vi "Generate Custom Error.vi"(8 "error in":errorcluster, 10 "PAR1":string, 11 "GOLPI error":T1) -> (0 "error out":errorcluster)   [LabVIEW 2020, in "GOLPI library.lvlib"]
doc: "Generate custom error of the GOLPI library. Some errors has input parameters (PAR1) to provide more detailed description."
uses:
  GOLPI library.lvlib
  Type Definitions/Custom Error Codes Enum Type Def.vi
  <vilib>/Utility/error.llb/Error Cluster From Error Code.vi
  <vilib>/ErrorRing/Error Ring.xnode
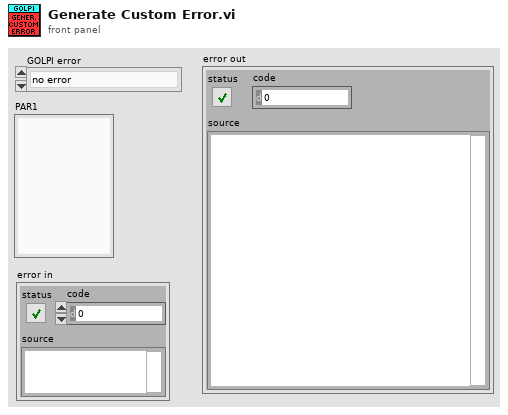
[diagram p1: front panel]
types:
  T1 = typedef "GOLPI library.lvlib/Custom Error Codes Enum Type Def.vi" = enum16{"no error", "00 working directory PAR1 missing", "01 octave binary PAR1 missing", "02 octave report error PAR1", "03 empty output last cmd PAR1", "04 missing temporary file PAR1", "05 pwd PAR 1 not exist", "06 oct package not installed", "07 octave default binary missing", "10 var PAR1 not string, vect", "11 var PAR1 not num, scal, ~compl", "12 var PAR1 not num, scal, compl", "13 var PAR1 not num, vect, ~compl", "14 var PAR1 not num, vect, compl", "15 var PAR1 not num, mat, ~compl", "16 var PAR1 not num, mat, ~compl", "30 read timeout", "60 bitstream transport failed", "61 bitstream decode error PAR1", "62 bitstream cannot be set", "70 struct transfer not possible", "80 struct: cluster elem. PAR1 not implem.", "81 struct: structure field PAR1 not implem.", "82 struct: size mismatch of PAR1", "83 struct: type mismatch of PAR1", "98 internal error", "99 not finished", "90 Not supported in Matlab mode", "91 Matlab variable transfer error", "92 Matlab Script Error", "100 Variable Pipe Mode cannot be set"}
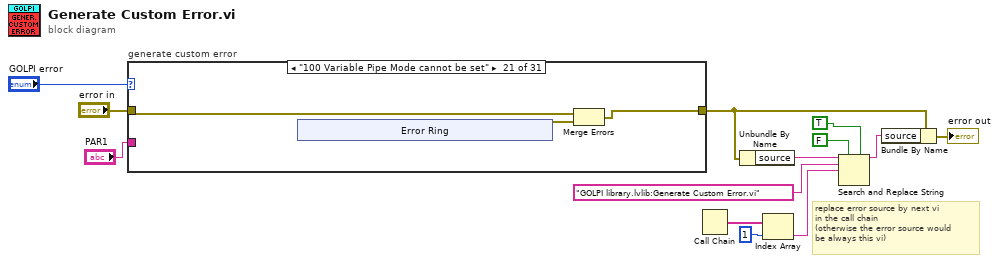
[diagram p0: block diagram]
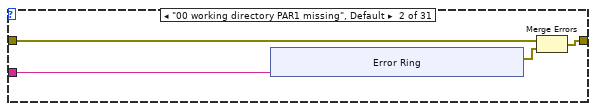
[diagram p3: hidden frame]
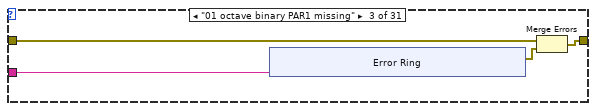
[diagram p4: hidden frame]
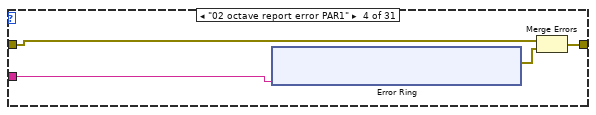
[diagram p5: hidden frame]
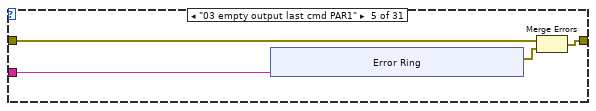
[diagram p6: hidden frame]
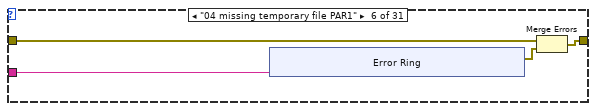
[diagram p7: hidden frame]
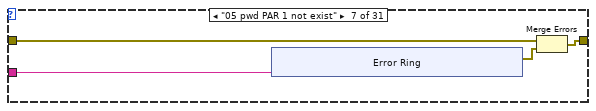
[diagram p8: hidden frame]
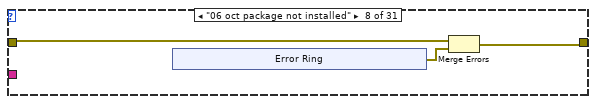
[diagram p9: hidden frame]
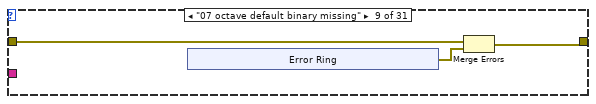
[diagram p10: hidden frame]
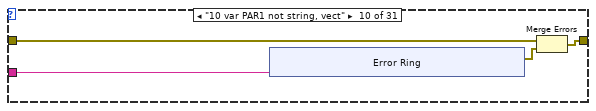
[diagram p11: hidden frame]
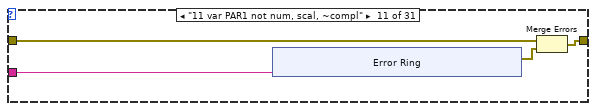
[diagram p12: hidden frame]
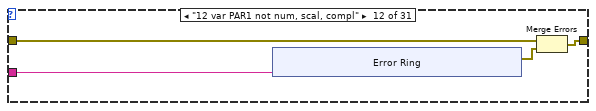
[diagram p13: hidden frame]
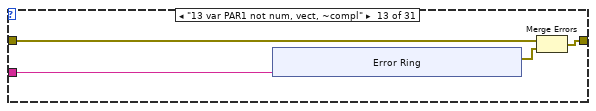
[diagram p14: hidden frame]
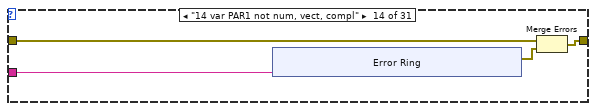
[diagram p15: hidden frame]
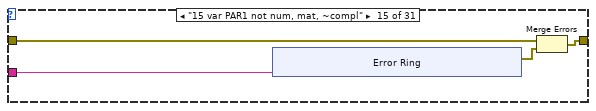
[diagram p16: hidden frame]
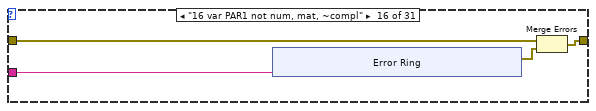
[diagram p17: hidden frame]
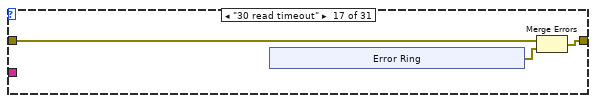
[diagram p18: hidden frame]
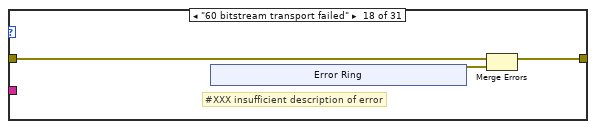
[diagram p19: hidden frame]
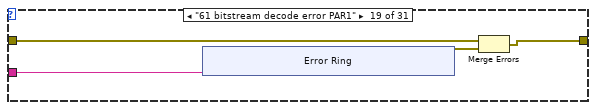
[diagram p20: hidden frame]
diagram:
  # "replace error source by next vi\nin the call chain\n(otherwise the error source would\nbe always this vi)"
  n1 = case "generate custom error" shown="\"100 Variable Pipe Mode cannot be set\"" "GOLPI error" {
    tunnel: "PAR1" -> [_ w18 w29 w38 w51 w59 w70 _ _ w97 w108 w120 w130 w142 w152 w163 _ _ w191 _ _ _ w225 w236 w247 w258 _ w277 w288 _ _]
    tunnel: [w14 w16 w27 w37 w48 w60 w71 w82 w89 w98 w109 w119 w132 w141 w153 w164 w174 w182 w192 w201 w209 w217 w226 w238 w249 w260 w270 w279 w290 w300 w307] -> w7
    tunnel: "error in" -> [w14 w15 w26 w39 w49 w61 w72 w81 w90 w99 w110 w122 w133 w143 w154 w165 w175 w183 w190 w202 w210 w218 w227 w237 w248 w259 w269 w278 w289 w299 w308]
    frame "no error" {
    }
    frame "00 working directory PAR1 missing", Default {
      n2 = xnode "Error Ring"("parameter 0"=w18) -> ("error out"=w17:errorcluster)
      n3 = Merge Errors(w15, w17) -> (w16:errorcluster)
    }
    frame "01 octave binary PAR1 missing" {
      n4 = xnode "Error Ring"("parameter 0"=w29) -> ("error out"=w28:errorcluster)
      n5 = Merge Errors(w26, w28) -> (w27:errorcluster)
    }
    frame "02 octave report error PAR1" {
      n6 = xnode "Error Ring"("parameter 0"=w38) -> ("error out"=w40:errorcluster)
      n7 = Merge Errors(w39, w40) -> (w37:errorcluster)
    }
    frame "03 empty output last cmd PAR1" {
      n8 = xnode "Error Ring"("parameter 0"=w51) -> ("error out"=w50:errorcluster)
      n9 = Merge Errors(w49, w50) -> (w48:errorcluster)
    }
    frame "04 missing temporary file PAR1" {
      n10 = xnode "Error Ring"("parameter 0"=w59) -> ("error out"=w62:errorcluster)
      n11 = Merge Errors(w61, w62) -> (w60:errorcluster)
    }
    frame "05 pwd PAR 1 not exist" {
      n12 = xnode "Error Ring"("parameter 0"=w70) -> ("error out"=w73:errorcluster)
      n13 = Merge Errors(w72, w73) -> (w71:errorcluster)
    }
    frame "06 oct package not installed" {
      n14 = xnode "Error Ring"() -> ("error out"=w83:errorcluster)
      n15 = Merge Errors(w81, w83) -> (w82:errorcluster)
    }
    frame "07 octave default binary missing" {
      n16 = xnode "Error Ring"() -> ("error out"=w91:errorcluster)
      n17 = Merge Errors(w90, w91) -> (w89:errorcluster)
    }
    frame "10 var PAR1 not string, vect" {
      n18 = xnode "Error Ring"("parameter 0"=w97) -> ("error out"=w100:errorcluster)
      n19 = Merge Errors(w99, w100) -> (w98:errorcluster)
    }
    frame "11 var PAR1 not num, scal, ~compl" {
      n20 = xnode "Error Ring"("parameter 0"=w108) -> ("error out"=w111:errorcluster)
      n21 = Merge Errors(w110, w111) -> (w109:errorcluster)
    }
    frame "12 var PAR1 not num, scal, compl" {
      n22 = xnode "Error Ring"("parameter 0"=w120) -> ("error out"=w121:errorcluster)
      n23 = Merge Errors(w122, w121) -> (w119:errorcluster)
    }
    frame "13 var PAR1 not num, vect, ~compl" {
      n24 = xnode "Error Ring"("parameter 0"=w130) -> ("error out"=w131:errorcluster)
      n25 = Merge Errors(w133, w131) -> (w132:errorcluster)
    }
    frame "14 var PAR1 not num, vect, compl" {
      n26 = xnode "Error Ring"("parameter 0"=w142) -> ("error out"=w144:errorcluster)
      n27 = Merge Errors(w143, w144) -> (w141:errorcluster)
    }
    frame "15 var PAR1 not num, mat, ~compl" {
      n28 = xnode "Error Ring"("parameter 0"=w152) -> ("error out"=w155:errorcluster)
      n29 = Merge Errors(w154, w155) -> (w153:errorcluster)
    }
    frame "16 var PAR1 not num, mat, ~compl" {
      n30 = xnode "Error Ring"("parameter 0"=w163) -> ("error out"=w166:errorcluster)
      n31 = Merge Errors(w165, w166) -> (w164:errorcluster)
    }
    frame "30 read timeout" {
      n32 = xnode "Error Ring"() -> ("error out"=w176:errorcluster)
      n33 = Merge Errors(w175, w176) -> (w174:errorcluster)
    }
    frame "60 bitstream transport failed" {
      # "#XXX insufficient description of error"
      n34 = xnode "Error Ring"() -> ("error out"=w184:errorcluster)
      n35 = Merge Errors(w183, w184) -> (w182:errorcluster)
    }
    frame "61 bitstream decode error PAR1" {
      n36 = xnode "Error Ring"("parameter 0"=w191) -> ("error out"=w193:errorcluster)
      n37 = Merge Errors(w190, w193) -> (w192:errorcluster)
    }
    frame "62 bitstream cannot be set" {
      n38 = xnode "Error Ring"() -> ("error out"=w203:errorcluster)
      n39 = Merge Errors(w202, w203) -> (w201:errorcluster)
    }
    frame "100 Variable Pipe Mode cannot be set" {
      n40 = xnode "Error Ring"() -> ("error out"=w211:errorcluster)
      n41 = Merge Errors(w210, w211) -> (w209:errorcluster)
    }
    frame "70 struct transfer not possible" {
      n42 = xnode "Error Ring"() -> ("error out"=w219:errorcluster)
      n43 = Merge Errors(w218, w219) -> (w217:errorcluster)
    }
    frame "80 struct: cluster elem. PAR1 not implem." {
      n44 = xnode "Error Ring"("parameter 0"=w225) -> ("error out"=w228:errorcluster)
      n45 = Merge Errors(w227, w228) -> (w226:errorcluster)
    }
    frame "81 struct: structure field PAR1 not implem." {
      n46 = xnode "Error Ring"("parameter 0"=w236) -> ("error out"=w239:errorcluster)
      n47 = Merge Errors(w237, w239) -> (w238:errorcluster)
    }
    frame "82 struct: size mismatch of PAR1" {
      n48 = xnode "Error Ring"("parameter 0"=w247) -> ("error out"=w250:errorcluster)
      n49 = Merge Errors(w248, w250) -> (w249:errorcluster)
    }
    frame "83 struct: type mismatch of PAR1" {
      n50 = xnode "Error Ring"("parameter 0"=w258) -> ("error out"=w261:errorcluster)
      n51 = Merge Errors(w259, w261) -> (w260:errorcluster)
    }
    frame "90 Not supported in Matlab mode" {
      n52 = xnode "Error Ring"() -> ("error out"=w271:errorcluster)
      n53 = Merge Errors(w269, w271) -> (w270:errorcluster)
    }
    frame "91 Matlab variable transfer error" {
      n54 = xnode "Error Ring"("parameter 0"=w277) -> ("error out"=w280:errorcluster)
      n55 = Merge Errors(w278, w280) -> (w279:errorcluster)
    }
    frame "92 Matlab Script Error" {
      n56 = xnode "Error Ring"("parameter 0"=w288) -> ("error out"=w291:errorcluster)
      n57 = Merge Errors(w289, w291) -> (w290:errorcluster)
    }
    frame "98 internal error" {
      n58 = xnode "Error Ring"() -> ("error out"=w301:errorcluster)
      n59 = Merge Errors(w299, w301) -> (w300:errorcluster)
    }
    frame "99 not finished" {
      n60 = xnode "Error Ring"() -> ("error out"=w309:errorcluster)
      n61 = Merge Errors(w308, w309) -> (w307:errorcluster)
    }
  }
  n62 = Call Chain() -> (call chain=w5:string[])
  n63 = Unbundle By Name(w7) -> ("source"=w9:string)
  n64 = Index Array(array=w5, index=1) -> (element=w3:string)
  n65 = Search and Replace String(replace all?=FALSE ("replace all? (F)"), multiline?=TRUE ("multiline? (F)"), input string=w9, search string="GOLPI library.lvlib:Generate Custom Error.vi", replace string=w3) -> (result string=w1:string)  [unwired: 3 in, 3 out]
  n66 = Bundle By Name(cluster=w7, "source"=w1) -> (→"error out":errorcluster)
